vi "S4GUI_001.vi"() -> ()   [LabVIEW 2018] (continued)
        n3587 = call "Read ASEL.vi"("error in (no error)"=w8930, "Instrument in"=w8931) -> ("error out"=w8927:errorcluster, "Opt_Selector.lvclass"=w8929:refnum<class "Opt_Selector.lvclass">, "Instrument out"=w8921:refnum<class "Instrument.lvclass">)  [unwired: 7 in]
        n3588 = call-dynamic "Read State Machine.vi"("error in (no error)"=w8927, "Device in"=w8929) -> ("error out"=w8926:errorcluster, "State Machine.lvclass"=w8915:refnum<class "State Machine.lvclass">, "Device out"=w8923:refnum<class "Opt_Selector.lvclass">)  [unwired: 7 in]
        n3589 = call "Next State.vi"("error in (no error)"=w8926, "New_State"=1, "State Machine in"=w8915) -> ("error out"=w8925:errorcluster, "State Machine out"=w8924:refnum<class "State Machine.lvclass">)  [unwired: 7 in]
        n3590 = call-dynamic "Write State Machine.vi"("error in (no error)"=w8925, "State Machine.lvclass"=w8924, "Device in"=w8923) -> ("error out"=w8920:errorcluster, "Device out"=w8922:refnum<class "Opt_Selector.lvclass">)  [unwired: 7 in]
        n3591 = call "Write ASEL.vi"("error in (no error)"=w8920, "Opt_Selector.lvclass"=w8922, "Instrument in"=w8921) -> ("error out"=w8917:errorcluster, "Instrument out"=w8919:refnum<class "Instrument.lvclass">)  [unwired: 7 in]
        n3592 = call "Write Instrument.lvclass.vi"("error in (no error)"=w8917, "Instrument.lvclass"=w8919, "S4ACS_GUI in"=w8918) -> ("error out"=w8916:errorcluster, "S4ACS_GUI out"=w8914:refnum<class "S4GUI.lvclass">)  [unwired: 7 in]
      }
      event "ASEL_stop": Value Change {
        n3593 = event-data() -> ()  [unwired: 1 in, 4 out]
        n3594 = call "Read Instrument.lvclass.vi"("error in (no error)"=w8952, "S4ACS_GUI in"=w8953) -> ("error out"=w8950:errorcluster, "Instrument.lvclass"=w8951:refnum<class "Instrument.lvclass">, "S4ACS_GUI out"=w8937:refnum<class "S4GUI.lvclass">)  [unwired: 7 in]
        n3595 = call "Read ASEL.vi"("error in (no error)"=w8950, "Instrument in"=w8951) -> ("error out"=w8946:errorcluster, "Opt_Selector.lvclass"=w8949:refnum<class "Opt_Selector.lvclass">, "Instrument out"=w8940:refnum<class "Instrument.lvclass">)  [unwired: 7 in]
        n3596 = call-dynamic "Read State Machine.vi"("error in (no error)"=w8946, "Device in"=w8949) -> ("error out"=w8945:errorcluster, "State Machine.lvclass"=w8948:refnum<class "State Machine.lvclass">, "Device out"=w8942:refnum<class "Opt_Selector.lvclass">)  [unwired: 7 in]
        n3597 = call "Next State.vi"("error in (no error)"=w8945, "New_State"=10, "State Machine in"=w8948) -> ("error out"=w8944:errorcluster, "State Machine out"=w8943:refnum<class "State Machine.lvclass">)  [unwired: 7 in]
        n3598 = call-dynamic "Write State Machine.vi"("error in (no error)"=w8944, "State Machine.lvclass"=w8943, "Device in"=w8942) -> ("error out"=w8939:errorcluster, "Device out"=w8941:refnum<class "Opt_Selector.lvclass">)  [unwired: 7 in]
        n3599 = call "Write ASEL.vi"("error in (no error)"=w8939, "Opt_Selector.lvclass"=w8941, "Instrument in"=w8940) -> ("error out"=w8936:errorcluster, "Instrument out"=w8938:refnum<class "Instrument.lvclass">)  [unwired: 7 in]
        n3600 = call "Write Instrument.lvclass.vi"("error in (no error)"=w8936, "Instrument.lvclass"=w8938, "S4ACS_GUI in"=w8937) -> ("error out"=w8935:errorcluster, "S4ACS_GUI out"=w8934:refnum<class "S4GUI.lvclass">)  [unwired: 7 in]
      }
      event "ASEL_init": Value Change {
        n3601 = event-data() -> ()  [unwired: 1 in, 4 out]
        n3602 = call "Read Instrument.lvclass.vi"("error in (no error)"=w8972, "S4ACS_GUI in"=w8973) -> ("error out"=w8970:errorcluster, "Instrument.lvclass"=w8971:refnum<class "Instrument.lvclass">, "S4ACS_GUI out"=w8957:refnum<class "S4GUI.lvclass">)  [unwired: 7 in]
        n3603 = call "Read ASEL.vi"("error in (no error)"=w8970, "Instrument in"=w8971) -> ("error out"=w8966:errorcluster, "Opt_Selector.lvclass"=w8969:refnum<class "Opt_Selector.lvclass">, "Instrument out"=w8960:refnum<class "Instrument.lvclass">)  [unwired: 7 in]
        n3604 = call-dynamic "Read State Machine.vi"("error in (no error)"=w8966, "Device in"=w8969) -> ("error out"=w8965:errorcluster, "State Machine.lvclass"=w8968:refnum<class "State Machine.lvclass">, "Device out"=w8962:refnum<class "Opt_Selector.lvclass">)  [unwired: 7 in]
        n3605 = call "Next State.vi"("error in (no error)"=w8965, "New_State"=30, "State Machine in"=w8968) -> ("error out"=w8964:errorcluster, "State Machine out"=w8963:refnum<class "State Machine.lvclass">)  [unwired: 7 in]
        n3606 = call-dynamic "Write State Machine.vi"("error in (no error)"=w8964, "State Machine.lvclass"=w8963, "Device in"=w8962) -> ("error out"=w8959:errorcluster, "Device out"=w8961:refnum<class "Opt_Selector.lvclass">)  [unwired: 7 in]
        n3607 = call "Write ASEL.vi"("error in (no error)"=w8959, "Opt_Selector.lvclass"=w8961, "Instrument in"=w8960) -> ("error out"=w8956:errorcluster, "Instrument out"=w8958:refnum<class "Instrument.lvclass">)  [unwired: 7 in]
        n3608 = call "Write Instrument.lvclass.vi"("error in (no error)"=w8956, "Instrument.lvclass"=w8958, "S4ACS_GUI in"=w8957) -> ("error out"=w8955:errorcluster, "S4ACS_GUI out"=w8954:refnum<class "S4GUI.lvclass">)  [unwired: 7 in]
      }
    }
    n3609 = flat-sequence {
      tunnel: w56 -> [w75]
      tunnel: w54 -> [w73]
      tunnel: [w75] -> w53
      tunnel: [w71] -> w52
      tunnel: [w70] -> w51
      tunnel: [w78] -> w55
      tunnel: w53 -> [w78]
      tunnel: w52 -> [w77]
      tunnel: w51 -> [w76]
      frame #0 {
        n3610 = Tick Count (ms)() -> (millisecond timer value=w74:u32)
        n3611 = local read "loop max(ms)"() -> (w69:u32)
        n3612 = Subtract(x=w74, y=w73) -> (x-y=w71:u32)
        n3613 = Greater?(x=w71, y=w69) -> (0:w72:bool)
        n3614 = Select(t=w71, s=w72, f=w69) -> (s? t:f=w70:u32)
      }
      frame #1 {
        "loop time(ms)" <- w77
        "loop max(ms)" <- w76
      }
    }
  }
  n3615 = stacked-sequence "INTERFACE" {
    frame #0 {
    }
    frame #1 {
    }
    frame #2 {
    }
    frame #3 {
    }
    frame #4 {
    }
    frame #5 {
    }
    frame #6 {
    }
    frame #7 {
    }
  }
  n3616 = disable-structure shown="Enabled" {
    frame Disabled {
      n3617 = Unbundle By Name() -> ("CALW State"=w8977:i32, "ASEL State"=w8976:i32, "GMIR State"=w8975:i32, "GFOC State"=w8974:i32)  [unwired: 1 in, 2 out]
      n3618 = Not Equal To 0?(x=w8977) -> ()  [unwired: 1 out]
      n3619 = Not Equal To 0?(x=w8976) -> ()  [unwired: 1 out]
      n3620 = Not Equal To 0?(x=w8975) -> ()  [unwired: 1 out]
      n3621 = Not Equal To 0?(x=w8974) -> ()  [unwired: 1 out]
    }
    frame Enabled {
    }
  }
  n3622 = call-dynamic "End.vi"("S4ACS_GUI in"=w27) -> ("error out"=→"error out":errorcluster)  [unwired: 9 in, 1 out]
